vi "obj_DataLog Live Tag Strings.vi"(0 "method":T1, 5 "offset/time":dbl, 7 "string in":string, 9 "tag index":i32, 11 "error in (no error)":errorcluster) -> (4 "time":dbl format="%<%H:%M:%S%2u\n%Y/%m/%d>T", 8 "string out":string, 10 "dup tag index":i32, 15 "error out":errorcluster)   [LabVIEW 2012]
doc: "Holds the most recently appended string and corresponding string log file offset values for the various string tags in the live database. Also spinlocks the requisite tag buffer read and write operations so as to prevent mismatch between this string buffer and the point buffer on reading. Used to quickly retrieve the last appended string and to reuse multiple successive copies of the same string."
uses:
  typedefs/t_DataLog Live Tag Strings Methods.ctl
  typedefs/t_DataLog Tag Info List Methods.ctl
  typedefs/t_DataLog Tag Hash Methods.ctl
  typedefs/t_DataLog Tag Buffers Methods.ctl
  typedefs/clusters/t_DataLog Point.ctl
  subvis/private/glb_DataLog Runtime Parameterisation.vi
  subvis/private/glb_DataLog MCVD.vi
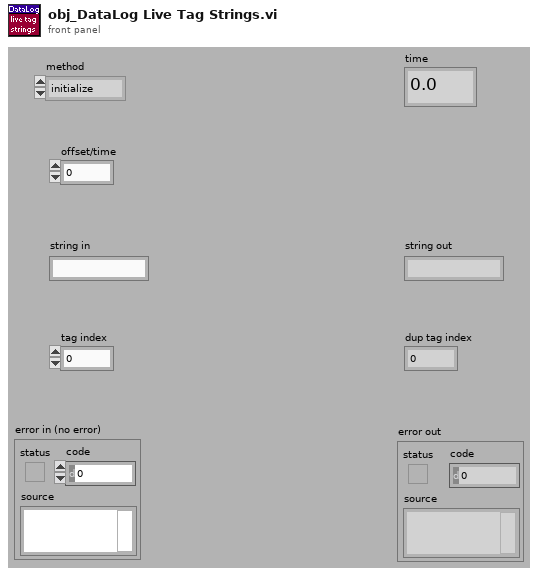
[diagram p1: front panel]
types:
  T1 = typedef "t_DataLog Live Tag Strings Methods.ctl" = enum16{"initialize", "rebuffer", "read", "write", "cleanup"}
  T2 = typedef "t_DataLog Tag Info List Methods.ctl" = enum16{"initialize", "create", "create empty", "rename", "delete", "test tag", "get", "get by name", "get default", "get list", "get path", "get subsets", "set subsets", "set config", "set capacity", "#tags", "go live", "set unlocked", "set mirrored"}
  T3 = typedef "t_DataLog Tag Hash Methods.ctl" = enum16{"initialize", "add tag", "index tag", "lookup", "#tags", "cleanup", "write recovery", "read recovery", "delete recovery"}
  T4 = typedef "t_DataLog Tag Buffers Methods.ctl" = enum16{"initialize", "inert", "write", "read", "read oldest", "read last", "cleanup"}
  T5 = typedef "t_DataLog Point.ctl" = cluster{"time":dbl, "value":dbl}
  T6 = typedef "t_DataLog Tag Config.ctl" = cluster{"name":string, "unit":string, "temporal":T7, "value":T8, "index":i32, "capacity":i32, "is meta?":bool, "mincapacity":i32, "deadband":dbl, "limit delay":dbl, "format":T9, "precision":u8, "undefine":bool, "update":bool, "update period":u16, "expression":string, "description":string, "logging algorithm":T10, "logging parameters":dbl[]}
  T7 = typedef "t_DataLog Temporal Types.ctl" = enum16{"set&hold", "sample", "event"}
  T8 = typedef "t_DataLog Value Types.ctl" = enum16{"number", "string"}
  T9 = typedef "t_DataLog Numerical Format.ctl" = enum8{"fractional", "exponential", "engineering"}
  T10 = typedef "t_DataLog Logging Algorithms.ctl" = enum16{"nothing", "changes", "everything", "every Nth", "time threshold", "value threshold + prior", "t or v threshold", "t or v threshold + prior"}
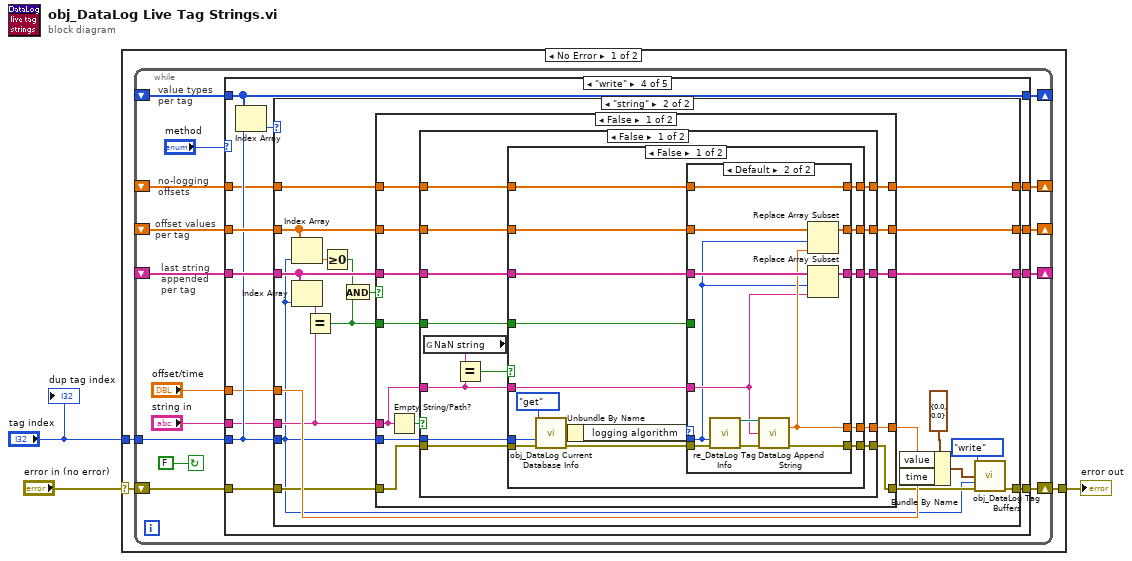
[diagram p0: block diagram]
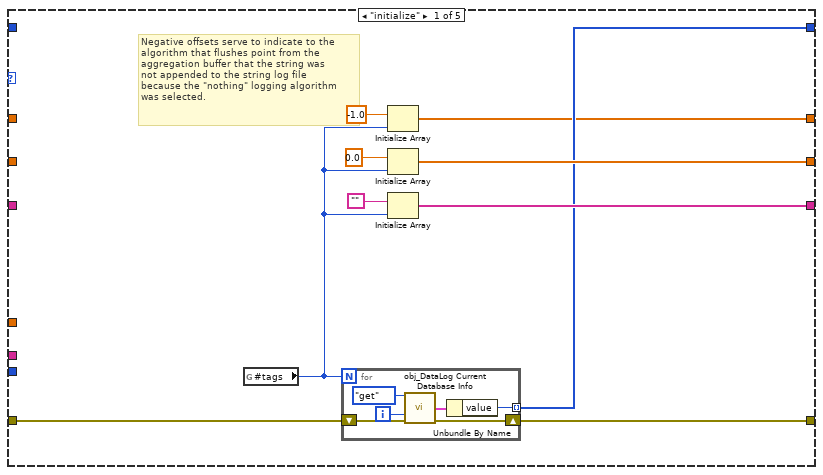
[diagram p2: hidden frame]
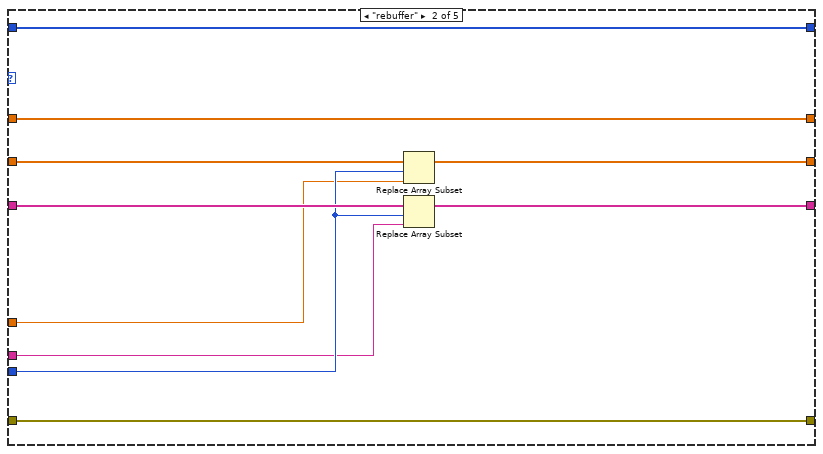
[diagram p3: hidden frame]
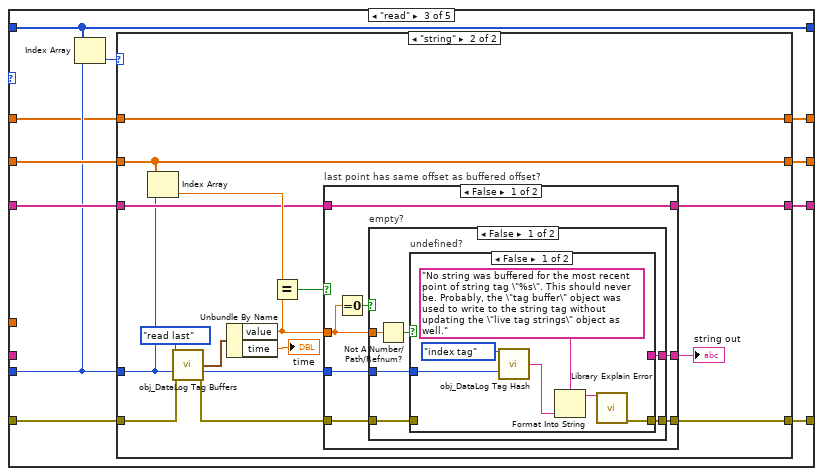
[diagram p4: hidden frame]
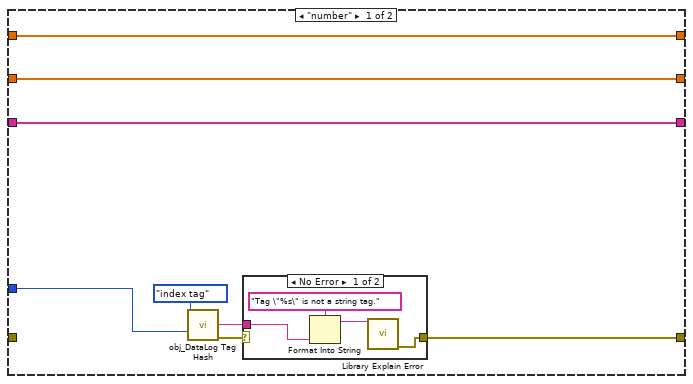
[diagram p5: hidden frame]
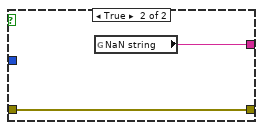
[diagram p7: hidden frame]
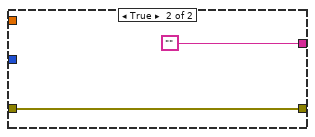
[diagram p8: hidden frame]
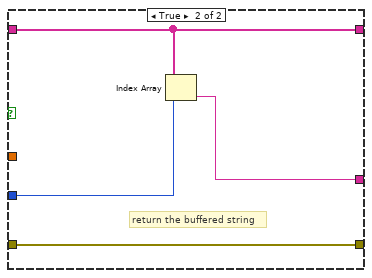
[diagram p9: hidden frame]
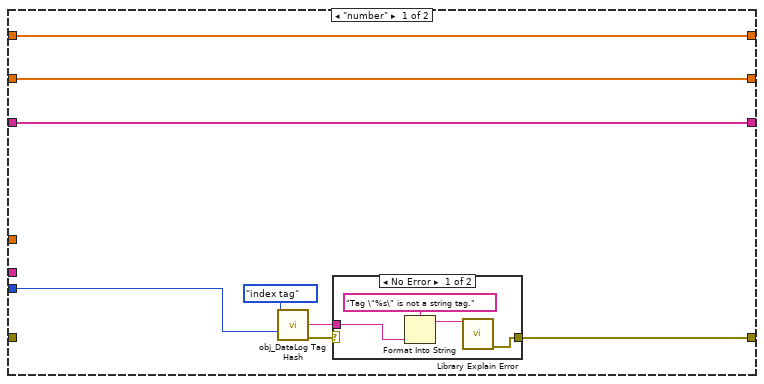
[diagram p10: hidden frame]
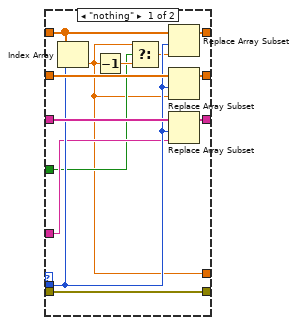
[diagram p12: hidden frame]
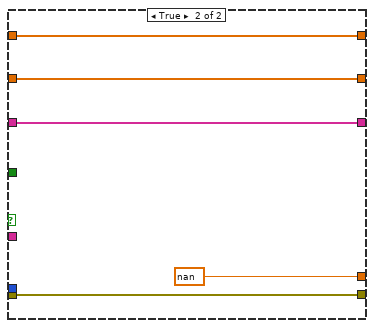
[diagram p13: hidden frame]
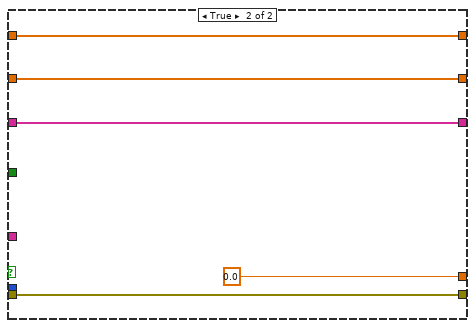
[diagram p14: hidden frame]
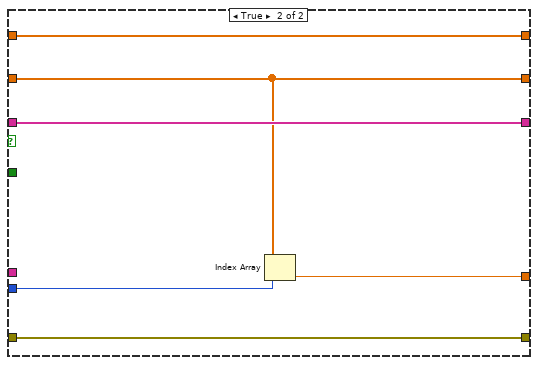
[diagram p15: hidden frame]
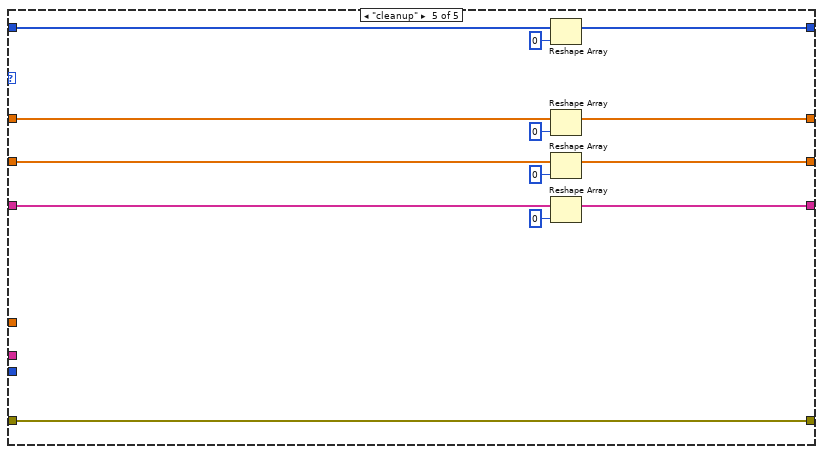
[diagram p16: hidden frame]
diagram:
  n1 = case shown="No Error" "error in (no error)" {
    selector: "error in (no error)" -> [w5 w260]
    tunnel: [w6 w260] -> w2
    tunnel: "tag index" -> [w4 _]
    frame No Error {
      n2 = while {
        shift-right: [w21] -> _
        shift-left: _ -> [w20]
        shift-right: [w19] -> w6
        shift-left: w5 -> [w18]
        shift-right: [w15] -> _
        shift-left: _ -> [w14]
        shift-right: [w13] -> _
        shift-left: _ -> [w12]
        tunnel: w4 -> [w9]
        shift-right: [w8] -> _
        shift-left: _ -> [w7]
        stop <- FALSE continue-if-true
        # "no-logging\noffsets"
        # "value types\nper tag"
        # "offset values\nper tag"
        # "last string\nappended\nper tag"
        n3 = case shown="\"write\"" "method" {
          tunnel: [w28 w46 w56 w125 w257] -> w21
          tunnel: w20 -> [_ w47 w57 w126 w258]
          tunnel: [w26 w42 w52 w121 w259] -> w19
          tunnel: w18 -> [w27 w42 w53 w122 w259]
          tunnel: [w31 w44 w54 w123 w253] -> w15
          tunnel: w14 -> [_ w45 w55 w124 w254]
          tunnel: [w25 w43 w50 w117 w250] -> w13
          tunnel: w12 -> [_ w43 w50 w117 w251]
          tunnel: "offset/time" -> [_ w40 _ w118 _]
          tunnel: "string in" -> [_ w39 _ w119 _]
          tunnel: w9 -> [_ w41 w51 w120 _]
          tunnel: [w23 w38 w48 w116 w247] -> w8
          tunnel: w7 -> [_ w38 w49 w115 w248]
          frame "initialize" {
            # "Negative offsets serve to indicate to the\nalgorithm that flushes point from the\naggregation buffer that the string was\nnot appended to the string log file\nbecause the \"nothing\" logging algorithm\nwas selected."
            n4 = global read "glb_DataLog Runtime Parameterisation.vi" "#tags"() -> (w22:i32)
            n5 = for {
              N: w22 -> [_]
              shift-right: [w33] -> w26
              shift-left: w27 -> [w34]
              tunnel: [w32] -> w25 mode=indexing
              i -> [w35]
              n6 = call "obj_DataLog Current Database Info.vi"("method"=t_DataLog_Tag_Info_List_Methods."get", "tag index/change#"=w35, "error in (no error)"=w34) -> ("tag config out"=w36:T6, "error out"=w33:errorcluster)  [unwired: 6 in, 5 out]
              n7 = Unbundle By Name(w36) -> ("value"=w32:T8)
            }
            n8 = Initialize Array(-1.0, w22) -> (w23:dbl[])
            n9 = Initialize Array(0.0, w22) -> (w28:dbl[])
            n10 = Initialize Array("", w22) -> (w31:string[])
          }
          frame "rebuffer" {
            n11 = Replace Array Subset(array=w47, new element=w40, index=w41) -> (w46:dbl[])
            n12 = Replace Array Subset(array=w45, new element=w39, index=w41) -> (w44:string[])
          }
          frame "read" {
            n13 = Index Array(array=w50, index=w51) -> (element=w58:T8)
            n14 = case shown="\"string\"" w58 {
              tunnel: w57 -> [w66 w87]
              tunnel: [w66 w87] -> w56
              tunnel: w55 -> [w65 w79]
              tunnel: [w65 w75] -> w54
              tunnel: w53 -> [_ w84]
              tunnel: [w61 w76] -> w52
              tunnel: w51 -> [w60 w74]
              tunnel: w49 -> [w59 w73]
              tunnel: [w59 w73] -> w48
              frame "number" {
                n15 = call "obj_DataLog Tag Hash.vi"("method"=t_DataLog_Tag_Hash_Methods."index tag", "tag index in"=w60) -> ("tag out"=w63:string, "error out"=w62:errorcluster)  [unwired: 10 in, 2 out]
                n16 = case shown="No Error" w62 {
                  selector: w62 -> [_ w71]
                  tunnel: [w70 w71] -> w61
                  tunnel: w63 -> [w69 _]
                  frame No Error {
                    n17 = Format Into String(format string="Tag \"%s\" is not a string tag.", w69) -> (resulting string=w67:string)  [unwired: 2 in, 1 out]
                    n18 = call "Library Explain Error.vi"("explanation prefix (none)"=w67) -> ("explained error"=w70:errorcluster)  [unwired: 14 in]
                  }
                  frame Error {
                  }
                }
              }
              frame "string" {
                n19 = Index Array(array=w87, index=w74) -> (element=w86:dbl)
                n20 = call "obj_DataLog Tag Buffers.vi"("method"=t_DataLog_Tag_Buffers_Methods."read last", "tag index"=w74, "error in (no error)"=w84) -> ("point out"=w83:T5, "tag index dup"=w77:i32, "error out"=w81:errorcluster)  [unwired: 8 in, 2 out]
                n21 = Unbundle By Name(w83) -> ("value"=w78:dbl, "time"=→"time":dbl)
                n22 = Equal?(x=w86, y=w78) -> (x = y?=w80:bool)
                n23 = case "last point has same offset as buffered offset?" shown="False" w80 {
                  tunnel: w78 -> [w93 _]
                  tunnel: w81 -> [w91 w114]
                  tunnel: w77 -> [w89 w113]
                  tunnel: [w92 w112] -> w72
                  tunnel: [w90 w114] -> w76
                  tunnel: w79 -> [w88 w111]
                  tunnel: [w88 w111] -> w75
                  frame False {
                    n24 = Equal To 0?(x=w93) -> (x = 0?=w94:bool)
                    n25 = case "empty?" shown="False" w94 {
                      tunnel: w93 -> [w100 _]
                      tunnel: [w98 ""] -> w92
                      tunnel: w91 -> [w96 w109]
                      tunnel: [w97 w109] -> w90
                      tunnel: w89 -> [w95 _]
                      frame False {
                        n26 = Not A Number/Path/Refnum?(number/path/refnum=w100) -> (NaN/Path/Refnum?=w99:bool)
                        n27 = case "undefined?" shown="False" w99 {
                          tunnel: [_ w108] -> w98
                          tunnel: [w102 w107] -> w97
                          tunnel: w96 -> [_ w107]
                          tunnel: w95 -> [w101 _]
                          frame False {
                            n28 = call "obj_DataLog Tag Hash.vi"("method"=t_DataLog_Tag_Hash_Methods."index tag", "tag index in"=w101) -> ("tag out"=w104:string)  [unwired: 10 in, 3 out]
                            n29 = Format Into String(format string="No string was buffered for the most recent point of string tag \"%s\". This should never be. Probably, the \"tag buffer\" object was used to write to the string tag without updating the \"live tag strings\" object as well.", w104) -> (resulting string=w106:string)  [unwired: 2 in, 1 out]
                            n30 = call "Library Explain Error.vi"("explanation prefix (none)"=w106) -> ("explained error"=w102:errorcluster)  [unwired: 14 in]
                          }
                          frame True {
                            n31 = global read "glb_DataLog MCVD.vi" "NaN string"() -> (w108:string)
                          }
                        }
                      }
                      frame True {
                      }
                    }
                  }
                  frame True {
                    # "return the buffered string"
                    n32 = Index Array(array=w111, index=w113) -> (element=w112:string)
                  }
                }
                "string out" <- w72
              }
            }
          }
          frame "write" {
            n33 = Index Array(array=w117, index=w120) -> (element=w127:T8)
            n34 = case shown="\"string\"" w127 {
              tunnel: w126 -> [w135 w146]
              tunnel: [w135 w152] -> w125
              tunnel: w124 -> [w134 w147]
              tunnel: [w134 w153] -> w123
              tunnel: w122 -> [_ w151]
              tunnel: [w129 w157] -> w121
              tunnel: w120 -> [w130 w145]
              tunnel: w119 -> [_ w155]
              tunnel: w118 -> [_ w156]
              tunnel: [w128 w149] -> w116
              tunnel: w115 -> [w128 w148]
              frame "number" {
                n35 = call "obj_DataLog Tag Hash.vi"("method"=t_DataLog_Tag_Hash_Methods."index tag", "tag index in"=w130) -> ("tag out"=w132:string, "error out"=w131:errorcluster)  [unwired: 10 in, 2 out]
                n36 = case shown="No Error" w131 {
                  selector: w131 -> [_ w140]
                  tunnel: [w139 w140] -> w129
                  tunnel: w132 -> [w138 _]
                  frame No Error {
                    n37 = Format Into String(format string="Tag \"%s\" is not a string tag.", w138) -> (resulting string=w136:string)  [unwired: 2 in, 1 out]
                    n38 = call "Library Explain Error.vi"("explanation prefix (none)"=w136) -> ("explained error"=w139:errorcluster)  [unwired: 14 in]
                  }
                  frame Error {
                  }
                }
              }
              frame "string" {
                n39 = Index Array(array=w146, index=w145) -> (element=w144:dbl)
                n40 = Index Array(array=w147, index=w145) -> (element=w161:string)
                n41 = Equal?(x=w161, y=w155) -> (x = y?=w141:bool)
                n42 = Greater Or Equal To 0?(x=w144) -> (x >= 0?=w143:bool)
                n43 = And(x=w143, y=w141) -> (x .and. y?=w142:bool)
                n44 = case shown="False" w142 {
                  tunnel: [w174 w245] -> w154
                  tunnel: w155 -> [w172 _]
                  tunnel: w145 -> [w171 w246]
                  tunnel: w146 -> [w168 w243]
                  tunnel: [w165 w244] -> w153
                  tunnel: w147 -> [w166 w244]
                  tunnel: [w167 w243] -> w152
                  tunnel: w151 -> [w170 w242]
                  tunnel: [w169 w242] -> w150
                  tunnel: [w164 w241] -> w149
                  tunnel: w148 -> [w163 w241]
                  tunnel: w141 -> [w162 _]
                  frame False {
                    n45 = Empty String/Path?(string/path=w172) -> (empty?=w173:bool)
                    n46 = case shown="False" w173 {
                      tunnel: w172 -> [w185 _]
                      tunnel: [w188 w239] -> w169
                      tunnel: [w187 0.0 ("offset")] -> w174
                      tunnel: w171 -> [w183 _]
                      tunnel: w170 -> [w182 w239]
                      tunnel: w168 -> [w181 w238]
                      tunnel: [w180 w238] -> w167
                      tunnel: w166 -> [w179 w237]
                      tunnel: [w178 w237] -> w165
                      tunnel: [w177 w236] -> w164
                      tunnel: w163 -> [w176 w236]
                      tunnel: w162 -> [w175 _]
                      frame False {
                        n47 = global read "glb_DataLog MCVD.vi" "NaN string"() -> (w186:string)
                        n48 = Equal?(x=w186, y=w185) -> (x = y?=w184:bool)
                        n49 = case shown="False" w184 {
                          tunnel: w182 -> [w197 w235]
                          tunnel: [w205 w235] -> w188
                          tunnel: [w202 nan ("offset")] -> w187
                          tunnel: w185 -> [w195 _]
                          tunnel: w183 -> [w196 _]
                          tunnel: w181 -> [w204 w233]
                          tunnel: [w200 w233] -> w180
                          tunnel: w179 -> [w203 w232]
                          tunnel: [w201 w232] -> w178
                          tunnel: [w193 w231] -> w177
                          tunnel: w176 -> [w199 w231]
                          tunnel: w175 -> [w189 _]
                          frame False {
                            n50 = call "obj_DataLog Current Database Info.vi"("method"=t_DataLog_Tag_Info_List_Methods."get", "tag index/change#"=w196, "error in (no error)"=w197) -> ("tag config out"=w194:T6, "dup tag index"=w191:i32, "error out"=w190:errorcluster)  [unwired: 6 in, 4 out]
                            n51 = Unbundle By Name(w194) -> ("logging algorithm"=w192:T10)
                            n52 = case shown="Default" w192 {
                              tunnel: [w216 w228] -> w205
                              tunnel: w204 -> [w215 w227]
                              tunnel: w203 -> [w214 w226]
                              tunnel: [w207 w225] -> w202
                              tunnel: [w212 w224] -> w201
                              tunnel: [w213 w223] -> w200
                              tunnel: w199 -> [w217 w221]
                              tunnel: w195 -> [w210 w222]
                              tunnel: [w218 w221] -> w193
                              tunnel: w191 -> [w211 w219]
                              tunnel: w190 -> [w216 w220]
                              tunnel: w189 -> [w208 _]
                              frame "nothing" {
                                n53 = Index Array(array=w217, index=w211) -> (element=w207:dbl)
                                n54 = Decrement(x=w207) -> (x-1=w209:dbl)
                                n55 = Select(t=w207, s=w208, f=w209) -> (s? t:f=w206:dbl)
                                n56 = Replace Array Subset(array=w217, new element=w206, index=w211) -> (w218:dbl[])
                                n57 = Replace Array Subset(array=w215, new element=w207, index=w211) -> (w213:dbl[])
                                n58 = Replace Array Subset(array=w214, new element=w210, index=w211) -> (w212:string[])
                              }
                              frame Default {
                                n59 = call "re_DataLog Tag Info.vi"("tag index (use tag)"=w219, "error in (no error)"=w220) -> ("tag log directory"=w230:path, "error out"=w229:errorcluster)  [unwired: 10 in, 2 out]
                                n60 = call "DataLog Append String.vi"("tag log directory"=w230, "string"=w222, "error in (no error)"=w229) -> ("offset"=w225:dbl, "error out"=w228:errorcluster)  [unwired: 9 in, 2 out]
                                n61 = Replace Array Subset(array=w227, new element=w225, index=w219) -> (w223:dbl[])
                                n62 = Replace Array Subset(array=w226, new element=w222, index=w219) -> (w224:string[])
                              }
                            }
                          }
                          frame True {
                          }
                        }
                      }
                      frame True {
                      }
                    }
                  }
                  frame True {
                    n63 = Index Array(array=w243, index=w246) -> (element=w245:dbl)
                  }
                }
                n64 = Bundle By Name(cluster=T5 {"time"=0.0, "value"=0.0} ("point"), "value"=w154, "time"=w156) -> (w158:T5)
                n65 = call "obj_DataLog Tag Buffers.vi"("method"=t_DataLog_Tag_Buffers_Methods."write", "point in"=w158, "tag index"=w145, "error in (no error)"=w150) -> ("error out"=w157:errorcluster)  [unwired: 7 in, 4 out]
              }
            }
          }
          frame "cleanup" {
            n66 = Reshape Array(w251, 0 ("dimension size")) -> (w250:T8[])
            n67 = Reshape Array(w248, 0 ("dimension size")) -> (w247:dbl[])
            n68 = Reshape Array(w258, 0 ("dimension size")) -> (w257:dbl[])
            n69 = Reshape Array(w254, 0 ("dimension size")) -> (w253:string[])
          }
        }
      }
    }
    frame Error {
    }
  }
  "error out" <- w2
  "dup tag index" <- "tag index"
